vi "FTW-Container-Object-Keys.vi"(0 "FTW-Container In":refnum<class "FTW-Container.lvclass">, 11 "error in":errorcluster) -> (4 "FTW-Container Out":refnum<class "FTW-Container.lvclass">, 6 "Object Keys":string[](array[string]), 15 "error out":errorcluster)   [LabVIEW 2015, in "FTW-Container.lvclass"]
uses:
  FTW-Container.lvclass
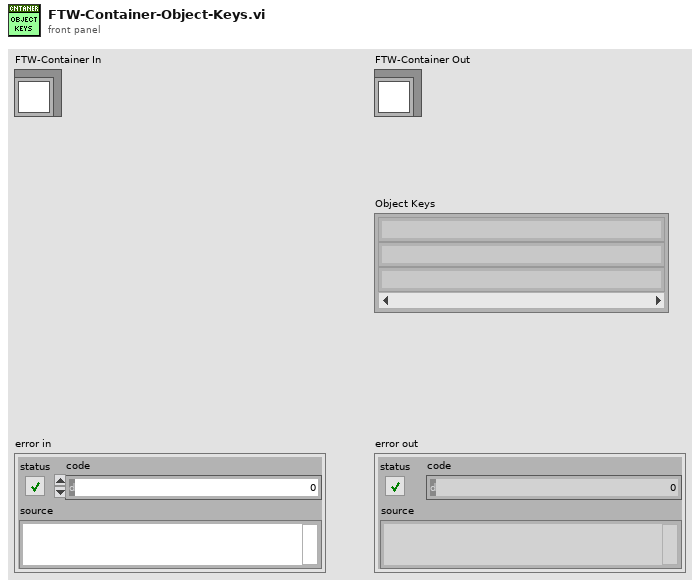
[diagram p1: front panel]
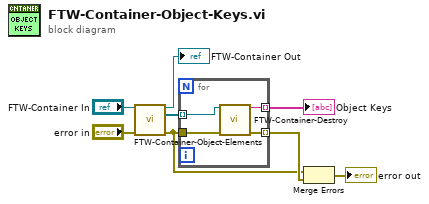
[diagram p0: block diagram]
diagram:
  n1 = call "FTW-Container-Object-Elements.vi"("FTW-Container In"="FTW-Container In", "error in"="error in") -> ("FTW-Container Out"=→"FTW-Container Out":refnum<class "FTW-Container.lvclass">, "Object Elements"=w2:refnum<class "FTW-Container.lvclass">[], "error out"=w3:errorcluster)  [unwired: 11 in]
  n2 = for {
    tunnel: w3 -> [w12]
    tunnel: [w11] -> w5 mode=indexing
    tunnel: w2 -> [w10] mode=indexing
    tunnel: [w9] -> w1 mode=indexing
    n3 = call "FTW-Container-Destroy.vi"("FTW-Container In"=w10, "error in"=w12) -> ("Name"=w9:string, "error out"=w11:errorcluster)  [unwired: 11 in, 1 out]
  }
  "Object Keys" <- w1
  n4 = Merge Errors(w3, w5) -> (→"error out":errorcluster)
